vi "CAPTH-Plot Several.vi"(0 "State":T1, 2 "Run List":string[](array[string])) -> (5 "Label":string, 6 "FINAL GRAPH":cluster{ext[], ext[]}[](graph))   [LabVIEW 2020]
uses:
  SUV/LV Source/SUV VIs/Typedefs/SUV-Experiment State.ctl
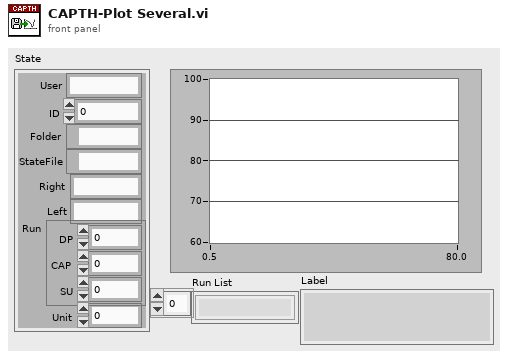
[diagram p1: front panel]
types:
  T1 = typedef "SUV-Experiment State.ctl" = cluster{"User":string, "ID":i32, "Folder":path, "Run":cluster{"DP":i32, "CAP":i32, "SU":i32}, "StateFile":path, "Right":string, "Left":string, "Unit":i32}
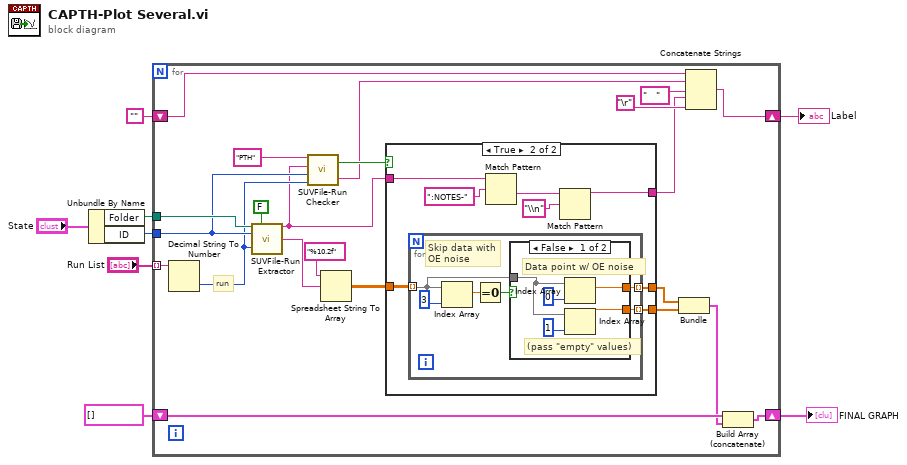
[diagram p0: block diagram]
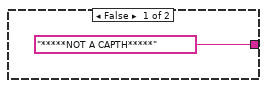
[diagram p2: hidden frame]
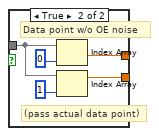
[diagram p3: hidden frame]
diagram:
  n1 = Unbundle By Name("State") -> ("Folder"=w4:path, "ID"=w5:i32)
  n2 = for {
    shift-right: [w29] -> w8
    shift-left: cluster{ext[], ext[]}[] [] -> [w28]
    tunnel: w5 -> [w24]
    tunnel: "Run List" -> [w26] mode=indexing
    tunnel: w4 -> [w27]
    shift-right: [w14] -> w1
    shift-left: "" -> [w9]
    # "run"
    n3 = Decimal String To Number(string=w26) -> (number=w23:i32)  [unwired: 2 in, 1 out]
    n4 = call "SUVFile-Run Extractor.vi"("Folder"=w27, "CAP (F) - SINGLE UNIT (T)"=FALSE, "Cat #"=w24, "Run #"=w23) -> ("HEADER STRING"=w13:string, "DATA STRING"=w17:string)  [unwired: 10 in]
    n5 = call "SUVFile-Run Checker.vi"("RUN #"=w23, "UNIT #"=w24, "HEADER INPUT"=w13, "STRING TO MATCH"="PTH") -> ("STRING \"UN-RN\""=w15:string, "OK"=w20:bool)
    n6 = Spreadsheet String To Array(format string="%10.2f", spreadsheet string=w17) -> (array=w12:dbl[][])  [unwired: 2 in]
    n7 = case shown="True" w20 {
      tunnel: w13 -> [_ w36]
      tunnel: ["*****NOT A CAPTH*****" w35] -> w16
      tunnel: w12 -> [_ w34]
      tunnel: [_ w33] -> w11
      tunnel: [_ w32] -> w10
      frame False {
      }
      frame True {
        n8 = for {
          tunnel: [w40] -> w32 mode=indexing
          tunnel: [w41] -> w33 mode=indexing
          tunnel: w34 -> [w42] mode=indexing
          # "Skip data with OE noise"
          n9 = Index Array(array=w42, index=3) -> (element=w44:dbl)
          n10 = Equal To 0?(x=w44) -> (x = 0?=w43:bool)
          n11 = case shown="False" w43 {
            tunnel: [w47 w51] -> w40
            tunnel: [w48 w52] -> w41
            tunnel: w42 -> [w46 w53]
            frame False {
              # "(pass \"empty\" values)"
              # "Data point w/ OE noise"
              n12 = Index Array(array=w46, index=0) -> (element=w48:dbl)
              n13 = Index Array(array=w46, index=1) -> (element=w47:dbl)
            }
            frame True {
              # "(pass actual data point)"
              # "Data point w/o OE noise"
              n14 = Index Array(array=w53, index=0) -> (element=w52:dbl)
              n15 = Index Array(array=w53, index=1) -> (element=w51:dbl)
            }
          }
        }
        n16 = Match Pattern(string=w36, regular expression=":NOTES-") -> (after substring=w38:string)  [unwired: 1 in, 3 out]
        n17 = Match Pattern(string=w38, regular expression="\\n") -> (before substring=w35:string)  [unwired: 1 in, 3 out]
      }
    }
    n18 = Bundle(w11, w10) -> (w21:cluster{dbl[], dbl[]})  [unwired: 1 in]
    n19 = Concatenate Strings(w9, w15, "   ", w16, "\r") -> (w14:string)
    n20 = Build Array (concatenate)(w28, w21) -> (w29:cluster{ext[], ext[]}[])
  }
  "FINAL GRAPH" <- w8
  "Label" <- w1
